vi "VoltageRatioInput Sensor Event Example.vi"() -> ()   [LabVIEW 2012, in "Phidget Voltage Ratio Input.lvlib"]
uses:
  <instrlib>/Phidgets/Phidget Voltage Ratio Input/Phidget Voltage Ratio Input.lvlib
  <instrlib>/Phidgets/Phidget Voltage Ratio Input/Public/VoltageRatioInputStart.vi
  <instrlib>/Phidgets/Phidget Voltage Ratio Input/Public/VoltageRatioInputClose.vi
  <instrlib>/Phidgets/Phidget Common/Phidget Common.lvlib
panel:
  in  "Sensor Type":u32(ring) items=["SENSOR_TYPE_VOLTAGERATIO"=0, "SENSOR_TYPE_1101_SHARP_2D120X"=11011, "SENSOR_TYPE_1101_SHARP_2Y0A21"=11012, "SENSOR_TYPE_1101_SHARP_2Y0A02"=11013, "SENSOR_TYPE_1102"=11020, "SENSOR_TYPE_1103"=11030, "SENSOR_TYPE_1104"=11040, "SENSOR_TYPE_1105"=11050, "SENSOR_TYPE_1106"=11060, "SENSOR_TYPE_1107"=11070, "SENSOR_TYPE_1108"=11080, "SENSOR_TYPE_1109"=11090, "SENSOR_TYPE_1110"=11100, "SENSOR_TYPE_1111"=11110, "SENSOR_TYPE_1112"=11120, "SENSOR_TYPE_1113"=11130, "SENSOR_TYPE_1115"=11150, "SENSOR_TYPE_1116"=11160, "SENSOR_TYPE_1118_AC"=11181, "SENSOR_TYPE_1118_DC"=11182, "SENSOR_TYPE_1119_AC"=11191, "SENSOR_TYPE_1119_DC"=11192, "SENSOR_TYPE_1120"=11200, "SENSOR_TYPE_1121"=11210, "SENSOR_TYPE_1122_AC"=11221, "SENSOR_TYPE_1122_DC"=11222, "SENSOR_TYPE_1124"=11240, "SENSOR_TYPE_1125_HUMIDITY"=11251, "SENSOR_TYPE_1125_TEMPERATURE"=11252, "SENSOR_TYPE_1126"=11260, "SENSOR_TYPE_1128"=11280, "SENSOR_TYPE_1129"=11290, "SENSOR_TYPE_1131"=11310, "SENSOR_TYPE_1134"=11340, "SENSOR_TYPE_1136"=11360, "SENSOR_TYPE_1137"=11370, "SENSOR_TYPE_1138"=11380, "SENSOR_TYPE_1139"=11390, "SENSOR_TYPE_1140"=11400, "SENSOR_TYPE_1141"=11410, "SENSOR_TYPE_1146"=11460, "SENSOR_TYPE_3120"=31200, "SENSOR_TYPE_3121"=31210, "SENSOR_TYPE_3122"=31220, "SENSOR_TYPE_3123"=31230, "SENSOR_TYPE_3130"=31300, "SENSOR_TYPE_3520"=35200, "SENSOR_TYPE_3521"=35210, "SENSOR_TYPE_3522"=35220]
  out "Unit Name":string
  out "Unit Symbol":string
  in  "IsHubPort":bool
  out "Sensor Value":dbl caption="Voltage Ratio" format="%.4f"
  in  "stop":bool
  out "Serial Number Return":i32
  in  "Device Info":T1={"Serial Number"=-1, "Channel"=0, "Port"=0}
  out "error out":errorcluster
  # "Be sure to use this stop button to stop the program.\nIf you use the \"Abort Execution\" button, you will\nneed to use PhidgetResetLibrary.vi or restart Labview \nin order for any Phidgets to work."
  # "Yes\n\nNo"
  # "Be sure to set sensor type to the sensor you're using.\nNo SensorChange events will fire using\nSENSOR_TYPE_VOLTAGERATIO"
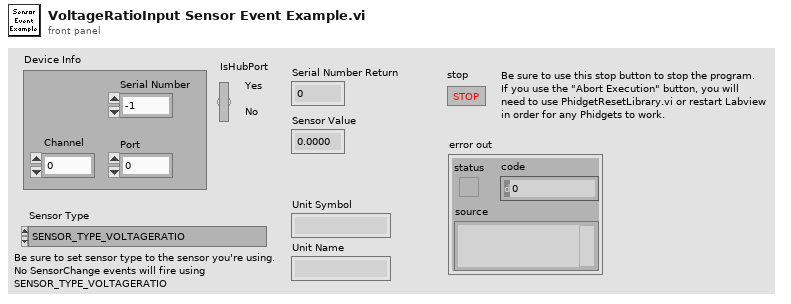
[diagram p1: front panel]
types:
  T1 = cluster{"Serial Number":i32, "Channel":i32, "Port":i32}
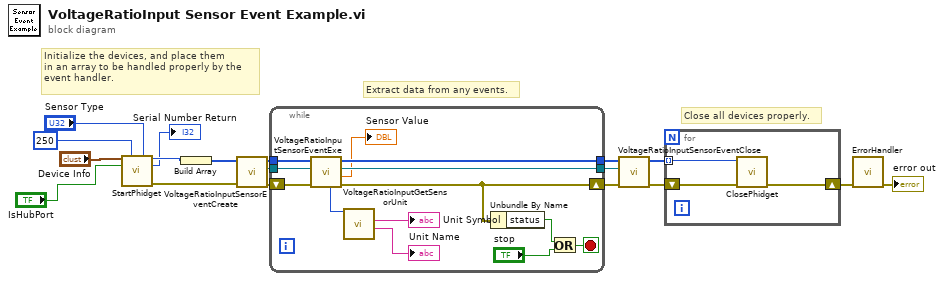
[diagram p0: block diagram]
diagram:
  # "Close all devices properly."
  # "Extract data from any events."
  # "Initialize the devices, and place them\nin an array to be handled properly by the\nevent handler."
  n1 = call-poly <instrlib>:"StartPhidget.vi"("Device Info"="Device Info", "Data Interval"=250, "Sesnor Type"="Sensor Type", "IsHubPort"="IsHubPort") -> ("Phidget ID"=w6:u64, "Serial Number Return"=→"Serial Number Return":i32, "error out"=w3:errorcluster)  [unwired: 8 in, 1 out]
  n2 = Build Array(w6) -> (w18:u64[])
  n3 = call <instrlib>:"VoltageRatioInputSensorEventCreate.vi"("error in (no error)"=w3, "Devices In"=w18) -> ("error out"=w11:errorcluster, "Event Registration Refnum"=w16:refnum<event-registration>, "Devices Out"=w17:u64[])  [unwired: 7 in]
  n4 = while {
    tunnel: w17 -> [w31]
    tunnel: w16 -> [w27]
    tunnel: [w30] -> w13
    shift-right: [w26] -> w12
    shift-left: w11 -> [w29]
    tunnel: [w28] -> w7
    stop <- w25 stop-if-true
    n5 = call <instrlib>:"VoltageRatioInputSensorEventExe.vi"("error in (no error)"=w29, "Event Registration Refnum In"=w27, "Devices In"=w31) -> ("error out"=w26:errorcluster, "Sensor Value"=→"Sensor Value":dbl, "Event Registration Refnum Out"=w30:refnum<event-registration>, "Devices Out"=w28:u64[], "phid"=w21:u64)  [unwired: 2 in, 2 out]
    n6 = call <instrlib>:"VoltageRatioInputGetSensorUnit.vi"("Device In"=w21) -> ("name"=→"Unit Name":string, "symbol"=→"Unit Symbol":string)  [unwired: 6 in, 2 out]
    n7 = Unbundle By Name(w26) -> ("status"=w23:bool)
    n8 = Or(x=w23, y="stop") -> (x .or. y?=w25:bool)
  }
  n9 = call <instrlib>:"VoltageRatioInputSensorEventClose.vi"("error in (no error)"=w12, "Event Registration Refnum In"=w13, "Devices In"=w7) -> ("error out"=w9:errorcluster, "Devices Out"=w8:u64[])  [unwired: 7 in]
  n10 = for {
    tunnel: w8 -> [w32] mode=indexing
    shift-right: [w34] -> w15
    shift-left: w9 -> [w33]
    n11 = call-poly <instrlib>:"ClosePhidget.vi"("error in"=w33, "Device In"=w32) -> ("error out"=w34:errorcluster)  [unwired: 9 in]
  }
  n12 = call <instrlib>:"ErrorHandler.vi"("error in"=w15) -> ("error out"=→"error out":errorcluster)  [unwired: 9 in, 1 out]
